vi "ReadTimeZoneCodes.vi"() -> (0 "x+y":dbl[](array[numeric])=[0.0, 1.0, 10.5, 9.5, -5.0, 10.5, 8.75, 3.0, -3.0, 11.0, 10.0, 11.0, 4.5, -8.0, -9.0, 6.0, -3.0, 5.0, -4.0, 4.0, 12.0, 12.0, 5.0, -3.0, 3.0, -4.0, -4.0, 9.0, 8.0, 0.0, -1.0, 5.0, 4.0, -12.0, 2.0, 8.0, -4.0, -2.0, -3.0, 6.0, 11.0, 1.0, 6.0, 3.0, 8.0, 2.0, 6.5, -5.0, -4.0, 2.0, 1.0, 13.75, 12.75, 9.0, 8.0, 8.0, 10.0, -4.0, -5.0, -10.0, -3.0, -3.0, -5.0, -6.0, 8.0, -5.0, -6.0, -1.0, 7.0, 10.0, 4.0, 7.0, 10.0, 5.0, -5.0, -5.0, 3.0, -5.0, -4.0, 3.0, 2.0, 0.0, -1.0, -5.0, -5.0, 6.0, 3.0, 13.0, 12.0, -3.0, -4.0, -2.0, 7.0, -6.0, -9.0, 4.0, -3.0, 12.0, 0.0, 4.0, -2.0, -4.0, 8.0, -9.0, -10.0, 8.0, 8.0, 7.0, 7.0, 9.0, 7.0, 3.0, 6.0, 4.5, 9.0, 8.0, 3.5, 5.5, 1.0, 2.0, 9.0, 10.0, 6.0, 11.0, 8.0, 7.0, 9.0, 4.0, 11.0, 11.0, 10.5, 14.0, 12.0, 12.0, 10.0, -8.5, 5.0, -6.0, 12.0, 6.5, 4.0, 3.0, -7.0, -7.0, 4.0, 5.0, 8.0, -1.0, 11.0, -1.5, 11.0, 7.0, 6.0, 5.75, 12.0, -2.5, -11.0, 13.0, 12.0, -2.0, 7.0, 6.0, 5.0, -3.0, -7.0, -5.0, 12.0, 12.0, 10.0, 13.0, 8.0, 5.0, -2.0, -3.0, 11.0, -8.0, -8.0, -8.0, 9.0, -3.0, -4.0, 8.5, 8.5, -4.0, 6.0, -5.0, 4.0, -3.0, -6.0, 10.0, 4.0, 2.0, 11.0, 4.0, 8.0, 11.0, -3.0, -11.0, 3.0, -7.0, -10.0, 5.0, 5.0, 13.0, 9.0, 5.0, 13.0, 12.0, -8.0, 9.0, 8.0, 8.0, 8.0, 0.0, -2.0, -3.0, 5.0, -9.0, -3.5, 11.0, 10.0, 6.0, 11.0, -10.0, 12.0, -3.0, 2.0, 1.0, 1.0, 0.0, 12.0, -2.0, -3.0, 7.0, 9.0, 8.0, 13.0, 1.0, 0.0, -11.0, -12.0, 10.0, 9.0, 10.0, 6.0, 5.0, 0.0], 1 "Abbreviation":string[](array[string])=["Abbreviation", "A", "ACDT", "ACST", "ACT", "ACT", "ACWST", "ADT", "ADT", "AEDT", "AEST", "AET", "AFT", "AKDT", "AKST", "ALMT", "AMST", "AMST", "AMT", "AMT", "ANAST", "ANAT", "AQTT", "ART", "AST", "AST", "AT", "AWDT", "AWST", "AZOST", "AZOT", "AZST", "AZT", "AoE", "B", "BNT", "BOT", "BRST", "BRT", "BST", "BST", "BST", "BTT", "C", "CAST", "CAT", "CCT", "CDT", "CDT", "CEST", "CET", "CHADT", "CHAST", "CHOST", "CHOST", "CHOT", "CHUT", "CIDST", "CIST", "CKT", "CLST", "CLT", "COT", "CST", "CST", "CST", "CT", "CVT", "CXT", "ChST", "D", "DAVT", "DDUT", "E", "EASST", "EAST", "EAT", "ECT", "EDT", "EEST", "EET", "EGST", "EGT", "EST", "ET", "F", "FET", "FJST", "FJT", "FKST", "FKT", "FNT", "G", "GALT", "GAMT", "GET", "GFT", "GILT", "GMT", "GST", "GST", "GYT", "H", "HADT", "HAST", "HKT", "HOVST", "HOVST", "HOVT", "I", "ICT", "IDT", "IOT", "IRDT", "IRKST", "IRKT", "IRST", "IST", "IST", "IST", "JST", "K", "KGT", "KOST", "KRAST", "KRAT", "KST", "KUYT", "L", "LHDT", "LHST", "LINT", "M", "MAGST", "MAGT", "MART", "MAWT", "MDT", "MHT", "MMT", "MSD", "MSK", "MST", "MT", "MUT", "MVT", "MYT", "N", "NCT", "NDT", "NFT", "NOVST", "NOVT", "NPT", "NRT", "NST", "NUT", "NZDT", "NZST", "O", "OMSST", "OMST", "ORAT", "P", "PDT", "PET", "PETST", "PETT", "PGT", "PHOT", "PHT", "PKT", "PMDT", "PMST", "PONT", "PST", "PST", "PT", "PWT", "PYST", "PYT", "PYT", "PYT", "Q", "QYZT", "R", "RET", "ROTT", "S", "SAKT", "SAMT", "SAST", "SBT", "SCT", "SGT", "SRET", "SRT", "SST", "SYOT", "T", "TAHT", "TFT", "TJT", "TKT", "TLT", "TMT", "TOT", "TVT", "U", "ULAST", "ULAST", "ULAT", "ULAT", "UTC", "UYST", "UYT", "UZT", "V", "VET", "VLAST", "VLAT", "VOST", "VUT", "W", "WAKT", "WARST", "WAST", "WAT", "WEST", "WET", "WFT", "WGST", "WGT", "WIB", "WIT", "WITA", "WST", "WST", "WT", "X", "Y", "YAKST", "YAKT", "YAPT", "YEKST", "YEKT", "Z"])   [LabVIEW 2015]
doc: "In order to Read and Write to any of the numerous pre-configured LabJack T7 Registers, the expected data type needs to be identified. This VI parses the T7 MODBUS Map (.json file), and searches the array to identify the Data Type expected for a desired Register. It also returns the Register Name. Like Registers are grouped in the Map list (e.g. AIN#(0:254)), so if a Selected Register is not exactly matched, a nearest neighbor is sought toward -Inf, and the values of the Nearest Likely Register are returned."
uses:
  <vilib>/regexp/Match Regular Expression.xnode
panel:
  out "UTC Offset.m":string[](array[string])=["", "00", "30", "30", "00", "30 / +9", "45", "00", "00", "00", "00", "00 / +10", "30", "00", "00", "00", "00", "00", "00", "00", "00", "00", "00", "00", "00", "00", "00 / -3", "00", "00", "00", "00", "00", "00", "00", "00", "00", "00", "00", "00", "00", "00", "00", "00", "00", "00", "00", "30", "00", "00", "00", "00", "45", "45", "00", "00 / +9", "00", "00", "00", "00", "00", "00", "00", "00", "00", "00", "00", "00 / -5", "00", "00", "00", "00", "00", "00", "00", "00", "00", "00", "00", "00", "00", "00", "00", "00", "00", "00 / -4", "00", "00", "00", "00", "00", "00", "00", "00", "00", "00", "00", "00", "00", "00", "00", "00", "00", "00", "00", "00", "00", "00", "00 / +8", "00", "00", "00", "00", "00", "30", "00", "00", "30", "30", "00", "00", "00", "00", "00", "00", "00", "00", "00", "00", "00", "00", "30", "00", "00", "00", "00", "30", "00", "00", "00", "30", "00", "00", "00", "00 / -6", "00", "00", "00", "00", "00", "30", "00", "00", "00", "45", "00", "30", "00", "00", "00", "00", "00", "00", "00", "00", "00", "00", "00", "00", "00", "00", "00", "00", "00", "00", "00", "00", "00", "00 / -7", "00", "00", "00", "30", "30", "00", "00", "00", "00", "00", "00", "00", "00", "00", "00", "00", "00", "00", "00", "00", "00", "00", "00", "00", "00", "00", "00", "00", "00", "00", "00", "00", "00 / +9", "00", "00 / +9", "", "00", "00", "00", "00", "30", "00", "00", "00", "00", "00", "00", "00", "00", "00", "00", "00", "00", "00", "00", "00", "00", "00", "00", "00", "00", "00", "00", "00", "00", "00", "00", "00", "00"]
  out "text":string="Abbreviation\tTime Zone Name\tLocation\tOffset ( x)\nA\tAlpha Time Zone\tMilitary\t1:00\nACDT\tAustralian Central Daylight Time  CDT – Central Daylight Time CDST – Central Daylight Savings Time\tAustralia\t10:30\nACST\tAustralian Central Standard Time  CST – Central Standard Time\tAustralia\t9:30\nACT\tAcre Time\tSouth America\t-5:00:00\nACT\tAustralian Central Time\tAustralia\t10:30 / +9:30\nACWST\tAustralian Central Western Standard Time\tAustralia\t8:45\nADT\tArabia Daylight Time  AST – Arabia Summer Time\tAsia\t3:00\nADT\tAtlantic Daylight Time  ADST – Atlantic Daylight Saving Time AST – Atlantic Summer Time  HAA – Heure Avancée de l'Atlantique (French)\tNorth America Atlantic\t-3:00:00\nAEDT\tAustralian Eastern Daylight Time  EDT – Eastern Daylight Time EDST – Eastern Daylight Saving Time\tAustralia Pacific\t11:00\nAEST\tAustralian Eastern Standard Time  EST – Eastern Standard Time AET – Australian Eastern Time\tAustralia\t10:00\nAET\tAustralian Eastern Time\tAustralia Pacific\t11:00 / +10:00\nAFT\tAfghanistan Time\tAsia\t4:30\nAKDT\tAlaska Daylight Time  ADST – Alaska Daylight Saving Time\tNorth America\t-8:00:00\nAKST\tAlaska Standard Time  AT – Alaska Time\tNorth America\t-9:00:00\nALMT\tAlma-Ata Time\tAsia\t6:00\nAMST\tAmazon Summer Time\tSouth America\t-3:00:00\nAMST\tArmenia Summer Time  AMDT – Armenia Daylight Time\tAsia\t5:00\nAMT\tAmazon Time\tSouth America\t-4:00:00\nAMT\tArmenia Time\tAsia\t4:00\nANAST\tAnadyr Summer Time\tAsia\t12:00\nANAT\tAnadyr Time\tAsia\t12:00\nAQTT\tAqtobe Time\tAsia\t5:00\nART\tArgentina Time\tAntarctica South America\t-3:00:00\nAST\tArabia Standard Time  AST – Arabic Standard Time AST – Al Manamah Standard Time\tAsia\t3:00\nAST\tAtlantic Standard Time  AT – Atlantic Time  AST – Tiempo Estándar del Atlántico (Spanish) HNA – Heure Normale de l'Atlantique (French)\tNorth America Atlantic Caribbean\t-4:00:00\nAT\tAtlantic Time\tNorth America Atlantic Caribbean\t-4:00 / -3:00\nAWDT\tAustralian Western Daylight Time  WDT – Western Daylight Time WST – Western Summer Time\tAustralia\t9:00\nAWST\tAustralian Western Standard Time  WST – Western Standard Time WAT – Western Australia Time\tAustralia\t8:00\nAZOST\tAzores Summer Time  AZODT – Azores Daylight Time\tAtlantic\t0:00\nAZOT\tAzores Time  AZOST – Azores Standard Time\tAtlantic\t-1:00:00\nAZST\tAzerbaijan Summer Time\tAsia\t5:00\nAZT\tAzerbaijan Time\tAsia\t4:00\nAoE\tAnywhere on Earth\tPacific\t-12:00:00\nB\tBravo Time Zone\tMilitary\t2:00\nBNT\tBrunei Darussalam Time  BDT – Brunei Time\tAsia\t8:00\nBOT\tBolivia Time\tSouth America\t-4:00:00\nBRST\tBrasília Summer Time  BST – Brazil Summer Time BST – Brazilian Summer Time\tSouth America\t-2:00:00\nBRT\tBrasília Time  BT – Brazil Time BT – Brazilian Time\tSouth America\t-3:00:00\nBST\tBangladesh Standard Time\tAsia\t6:00\nBST\tBougainville Standard Time\tPacific\t11:00\nBST\tBritish Summer Time  BDT – British Daylight Time BDST – British Daylight Saving Time\tEurope\t1:00\nBTT\tBhutan Time\tAsia\t6:00\nC\tCharlie Time Zone\tMilitary\t3:00\nCAST\tCasey Time\tAntarctica\t8:00\nCAT\tCentral Africa Time\tAfrica\t2:00\nCCT\tCocos Islands Time\tIndian Ocean\t6:30\nCDT\tCentral Daylight Time  CDST – Central Daylight Saving Time NACDT – North American Central Daylight Time  HAC – Heure Avancée du Centre (French)\tNorth America\t-5:00:00\nCDT\tCuba Daylight Time\tCaribbean\t-4:00:00\nCEST\tCentral European Summer Time  CEDT – Central European Daylight Time ECST – European Central Summer Time  MESZ – Mitteleuropäische Sommerzeit (German)\tEurope Antarctica\t2:00\nCET\tCentral European Time  ECT – European Central Time CET – Central Europe Time  MEZ – Mitteleuropäische Zeit (German)\tEurope Africa Antarctica\t1:00\nCHADT\tChatham Island Daylight Time  CDT – Chatham Daylight Time\tPacific\t13:45\nCHAST\tChatham Island Standard Time\tPacific\t12:45\nCHOST\tChoibalsan Summer Time  CHODT – Choibalsan Daylight Time CHODST – Choibalsan Daylight Saving Time\tAsia\t9:00\nCHOST\tChoibalsan Summer Time\tAsia\t8:00 / +9:00\nCHOT\tChoibalsan Time\tAsia\t8:00\nCHUT\tChuuk Time\tPacific\t10:00\nCIDST\tCayman Islands Daylight Saving Time\tCaribbean\t-4:00:00\nCIST\tCayman Islands Standard Time  CIT – Cayman Islands Time\tCaribbean\t-5:00:00\nCKT\tCook Island Time\tPacific\t-10:00:00\nCLST\tChile Summer Time  CLDT – Chile Daylight Time\tSouth America Antarctica\t-3:00:00\nCLT\tChile Standard Time  CT – Chile Time CLST – Chile Standard Time\tSouth America Antarctica\t-3:00:00\nCOT\tColombia Time\tSouth America\t-5:00:00\nCST\tCentral Standard Time  CT – Central Time NACST – North American Central Standard Time  CST – Tiempo Central Estándar (Spanish) HNC – Heure Normale du Centre (French)\tNorth America Central America\t-6:00:00\nCST\tChina Standard Time\tAsia\t8:00\nCST\tCuba Standard Time\tCaribbean\t-5:00:00\nCT\tCentral Time\tNorth America Central America\t-6:00 / -5:00\nCVT\tCape Verde Time\tAfrica\t-1:00:00\nCXT\tChristmas Island Time\tAustralia\t7:00\nChST\tChamorro Standard Time  GST – Guam Standard Time\tPacific\t10:00\nD\tDelta Time Zone\tMilitary\t4:00\nDAVT\tDavis Time\tAntarctica\t7:00\nDDUT\tDumont-d'Urville Time\tAntarctica\t10:00\nE\tEcho Time Zone\tMilitary\t5:00\nEASST\tEaster Island Summer Time  EADT – Easter Island Daylight Time\tPacific\t-5:00:00\nEAST\tEaster Island Standard Time\tPacific\t-5:00:00\nEAT\tEastern Africa Time  EAT – East Africa Time\tAfrica Indian Ocean\t3:00\nECT\tEcuador Time\tSouth America\t-5:00:00\nEDT\tEastern Daylight Time  EDST – Eastern Daylight Savings Time NAEDT – North American Eastern Daylight Time  HAE – Heure Avancée de l'Est (French) EDT – Tiempo de verano del Este (Spanish)\tNorth America Caribbean\t-4:00:00\nEEST\tEastern European Summer Time  EEDT – Eastern European Daylight Time  OESZ – Osteuropäische Sommerzeit (German)\tEurope Asia\t3:00\nEET\tEastern European Time  OEZ – Osteuropäische Zeit (German)\tEurope Asia Africa\t2:00\nEGST\tEastern Greenland Summer Time  EGST – East Greenland Summer Time\tNorth America\t0:00\nEGT\tEast Greenland Time  EGT – Eastern Greenland Time\tNorth America\t-1:00:00\nEST\tEastern Standard Time  ET – Eastern Time  NAEST – North American Eastern Standard Time  ET – Tiempo del Este (Spanish) HNE – Heure Normale de l'Est (French)\tNorth America Caribbean Central America\t-5:00:00\nET\tEastern Time\tNorth America Caribbean Central America\t-5:00 / -4:00\nF\tFoxtrot Time Zone\tMilitary\t6:00\nFET\tFurther-Eastern European Time\tEurope\t3:00\nFJST\tFiji Summer Time  FJDT – Fiji Daylight Time\tPacific\t13:00\nFJT\tFiji Time\tPacific\t12:00\nFKST\tFalkland Islands Summer Time  FKDT – Falkland Island Daylight Time\tSouth America\t-3:00:00\nFKT\tFalkland Island Time  FKST – Falkland Island Standard Time\tSouth America\t-4:00:00\nFNT\tFernando de Noronha Time\tSouth America\t-2:00:00\nG\tGolf Time Zone\tMilitary\t7:00\nGALT\tGalapagos Time\tPacific\t-6:00:00\nGAMT\tGambier Time  GAMT – Gambier Islands Time\tPacific\t-9:00:00\nGET\tGeorgia Standard Time\tAsia\t4:00\nGFT\tFrench Guiana Time\tSouth America\t-3:00:00\nGILT\tGilbert Island Time\tPacific\t12:00\nGMT\tGreenwich Mean Time  \"– Coordinated Universal Time GT – Greenwich Time\tEurope Africa North America Antarctica\t0:00\nGST\tGulf Standard Time\tAsia\t4:00\nGST\tSouth Georgia Time\tSouth America\t-2:00:00\nGYT\tGuyana Time\tSouth America\t-4:00:00\nH\tHotel Time Zone\tMilitary\t8:00\nHADT\tHawaii-Aleutian Daylight Time  HDT – Hawaii Daylight Time\tNorth America\t-9:00:00\nHAST\tHawaii-Aleutian Standard Time  HST – Hawaii Standard Time\tNorth America Pacific\t-10:00:00\nHKT\tHong Kong Time\tAsia\t8:00\nHOVST\tHovd Summer Time  HOVDT – Hovd Daylight Time HOVDST – Hovd Daylight Saving Time\tAsia\t8:00\nHOVST\tHovd Summer Time\tAsia\t7:00 / +8:00\nHOVT\tHovd Time\tAsia\t7:00\nI\tIndia Time Zone\tMilitary\t9:00\nICT\tIndochina Time\tAsia\t7:00\nIDT\tIsrael Daylight Time\tAsia\t3:00\nIOT\tIndian Chagos Time\tIndian Ocean\t6:00\nIRDT\tIran Daylight Time  IRST – Iran Summer Time IDT – Iran Daylight Time\tAsia\t4:30\nIRKST\tIrkutsk Summer Time\tAsia\t9:00\nIRKT\tIrkutsk Time\tAsia\t8:00\nIRST\tIran Standard Time  IT – Iran Time\tAsia\t3:30\nIST\tIndia Standard Time  IT – India Time IST – Indian Standard Time\tAsia\t5:30\nIST\tIrish Standard Time  IST – Irish Summer Time\tEurope\t1:00\nIST\tIsrael Standard Time\tAsia\t2:00\nJST\tJapan Standard Time\tAsia\t9:00\nK\tKilo Time Zone\tMilitary\t10:00\nKGT\tKyrgyzstan Time\tAsia\t6:00\nKOST\tKosrae Time\tPacific\t11:00\nKRAST\tKrasnoyarsk Summer Time\tAsia\t8:00\nKRAT\tKrasnoyarsk Time\tAsia\t7:00\nKST\tKorea Standard Time  KST – Korean Standard Time KT – Korea Time\tAsia\t9:00\nKUYT\tKuybyshev Time  SAMST – Samara Summer Time\tEurope\t4:00\nL\tLima Time Zone\tMilitary\t11:00\nLHDT\tLord Howe Daylight Time\tAustralia\t11:00\nLHST\tLord Howe Standard Time\tAustralia\t10:30\nLINT\tLine Islands Time\tPacific\t14:00\nM\tMike Time Zone\tMilitary\t12:00\nMAGST\tMagadan Summer Time  MAGST – Magadan Island Summer Time\tAsia\t12:00\nMAGT\tMagadan Time  MAGT – Magadan Island Time\tAsia\t10:00\nMART\tMarquesas Time\tPacific\t-9:30:00\nMAWT\tMawson Time\tAntarctica\t5:00\nMDT\tMountain Daylight Time  MDST – Mountain Daylight Saving Time NAMDT – North American Mountain Daylight Time  HAR – Heure Avancée des Rocheuses (French)\tNorth America\t-6:00:00\nMHT\tMarshall Islands Time\tPacific\t12:00\nMMT\tMyanmar Time\tAsia\t6:30\nMSD\tMoscow Daylight Time  Moscow Summer Time\tEurope\t4:00\nMSK\tMoscow Standard Time  MCK – Moscow Time\tEurope Asia\t3:00\nMST\tMountain Standard Time  MT – Mountain Time NAMST – North American Mountain Standard Time  HNR – Heure Normale des Rocheuses (French)\tNorth America\t-7:00:00\nMT\tMountain Time\tNorth America\t-7:00 / -6:00\nMUT\tMauritius Time\tAfrica\t4:00\nMVT\tMaldives Time\tAsia\t5:00\nMYT\tMalaysia Time  MST – Malaysian Standard Time\tAsia\t8:00\nN\tNovember Time Zone\tMilitary\t-1:00:00\nNCT\tNew Caledonia Time\tPacific\t11:00\nNDT\tNewfoundland Daylight Time  HAT – Heure Avancée de Terre-Neuve (French)\tNorth America\t-2:30:00\nNFT\tNorfolk Time  NFT – Norfolk Island Time\tAustralia\t11:00\nNOVST\tNovosibirsk Summer Time  OMSST – Omsk Summer Time\tAsia\t7:00\nNOVT\tNovosibirsk Time  OMST – Omsk Standard Time\tAsia\t6:00\nNPT\tNepal Time\tAsia\t5:45\nNRT\tNauru Time\tPacific\t12:00\nNST\tNewfoundland Standard Time  HNT – Heure Normale de Terre-Neuve (French)\tNorth America\t-3:30:00\nNUT\tNiue Time\tPacific\t-11:00:00\nNZDT\tNew Zealand Daylight Time\tPacific Antarctica\t13:00\nNZST\tNew Zealand Standard Time\tPacific Antarctica\t12:00\nO\tOscar Time Zone\tMilitary\t-2:00:00\nOMSST\tOmsk Summer Time  NOVST – Novosibirsk Summer Time\tAsia\t7:00\nOMST\tOmsk Standard Time  OMST – Omsk Time NOVT – Novosibirsk Time\tAsia\t6:00\nORAT\tOral Time\tAsia\t5:00\nP\tPapa Time Zone\tMilitary\t-3:00:00\nPDT\tPacific Daylight Time  PDST – Pacific Daylight Saving Time NAPDT – North American Pacific Daylight Time  HAP – Heure Avancée du Pacifique (French)\tNorth America\t-7:00:00\nPET\tPeru Time\tSouth America\t-5:00:00\nPETST\tKamchatka Summer Time\tAsia\t12:00\nPETT\tKamchatka Time  PETT – Petropavlovsk-Kamchatski Time\tAsia\t12:00\nPGT\tPapua New Guinea Time\tPacific\t10:00\nPHOT\tPhoenix Island Time\tPacific\t13:00\nPHT\tPhilippine Time  PST – Philippine Standard Time\tAsia\t8:00\nPKT\tPakistan Standard Time  PKT – Pakistan Time\tAsia\t5:00\nPMDT\tPierre & Miquelon Daylight Time\tNorth America\t-2:00:00\nPMST\tPierre & Miquelon Standard Time\tNorth America\t-3:00:00\nPONT\tPohnpei Standard Time\tPacific\t11:00\nPST\tPacific Standard Time  PT – Pacific Time NAPST – North American Pacific Standard Time  PT – Tiempo del Pacífico (Spanish) HNP – Heure Normale du Pacifique (French)\tNorth America\t-8:00:00\nPST\tPitcairn Standard Time\tPacific\t-8:00:00\nPT\tPacific Time\tNorth America\t-8:00 / -7:00\nPWT\tPalau Time\tPacific\t9:00\nPYST\tParaguay Summer Time\tSouth America\t-3:00:00\nPYT\tParaguay Time\tSouth America\t-4:00:00\nPYT\tPyongyang Time  PYST – Pyongyang Standard Time\tAsia\t8:30\nPYT\tPyongyang Time\tAsia\t8:30\nQ\tQuebec Time Zone\tMilitary\t-4:00:00\nQYZT\tQyzylorda Time\tAsia\t6:00\nR\tRomeo Time Zone\tMilitary\t-5:00:00\nRET\tReunion Time\tAfrica\t4:00\nROTT\tRothera Time\tAntarctica\t-3:00:00\nS\tSierra Time Zone\tMilitary\t-6:00:00\nSAKT\tSakhalin Time\tAsia\t10:00\nSAMT\tSamara Time  SAMT – Samara Standard Time\tEurope\t4:00\nSAST\tSouth Africa Standard Time  SAST – South African Standard Time\tAfrica\t2:00\nSBT\tSolomon Islands Time  SBT – Solomon Island Time\tPacific\t11:00\nSCT\tSeychelles Time\tAfrica\t4:00\nSGT\tSingapore Time  SST – Singapore Standard Time\tAsia\t8:00\nSRET\tSrednekolymsk Time\tAsia\t11:00\nSRT\tSuriname Time\tSouth America\t-3:00:00\nSST\tSamoa Standard Time\tPacific\t-11:00:00\nSYOT\tSyowa Time\tAntarctica\t3:00\nT\tTango Time Zone\tMilitary\t-7:00:00\nTAHT\tTahiti Time\tPacific\t-10:00:00\nTFT\tFrench Southern and Antarctic Time  KIT – Kerguelen (Islands) Time\tIndian Ocean\t5:00\nTJT\tTajikistan Time\tAsia\t5:00\nTKT\tTokelau Time\tPacific\t13:00\nTLT\tEast Timor Time\tAsia\t9:00\nTMT\tTurkmenistan Time\tAsia\t5:00\nTOT\tTonga Time\tPacific\t13:00\nTVT\tTuvalu Time\tPacific\t12:00\nU\tUniform Time Zone\tMilitary\t-8:00:00\nULAST\tUlaanbaatar Summer Time  ULAST – Ulan Bator Summer Time\tAsia\t9:00\nULAST\tUlaanbaatar Summer Time\tAsia\t8:00 / +9:00\nULAT\tUlaanbaatar Time  ULAT – Ulan Bator Time\tAsia\t8:00\nULAT\tUlaanbaatar Time\tAsia\t8:00 / +9:00\nUTC\tCoordinated Universal Time\tWorldwide\tUTC\nUYST\tUruguay Summer Time\tSouth America\t-2:00:00\nUYT\tUruguay Time\tSouth America\t-3:00:00\nUZT\tUzbekistan Time\tAsia\t5:00\nV\tVictor Time Zone\tMilitary\t-9:00:00\nVET\tVenezuelan Standard Time  HLV – Hora Legal de Venezuela (Spanish)\tSouth America\t-4:30:00\nVLAST\tVladivostok Summer Time\tAsia\t11:00\nVLAT\tVladivostok Time\tAsia\t10:00\nVOST\tVostok Time\tAntarctica\t6:00\nVUT\tVanuatu Time  EFATE – Efate Time\tPacific\t11:00\nW\tWhiskey Time Zone\tMilitary\t-10:00:00\nWAKT\tWake Time\tPacific\t12:00\nWARST\tWestern Argentine Summer Time\tSouth America\t-3:00:00\nWAST\tWest Africa Summer Time\tAfrica\t2:00\nWAT\tWest Africa Time\tAfrica\t1:00\nWEST\tWestern European Summer Time  WEDT – Western European Daylight Time  WESZ – Westeuropäische Sommerzeit (German)\tEurope Africa\t1:00\nWET\tWestern European Time  GMT – Greenwich Mean Time  WEZ – Westeuropäische Zeit (German)\tEurope Africa\t0:00\nWFT\tWallis and Futuna Time\tPacific\t12:00\nWGST\tWestern Greenland Summer Time  WGST – West Greenland Summer Time\tNorth America\t-2:00:00\nWGT\tWest Greenland Time  WGT – Western Greenland Time\tNorth America\t-3:00:00\nWIB\tWestern Indonesian Time  WIB – Waktu Indonesia Barat\tAsia\t7:00\nWIT\tEastern Indonesian Time  WIT – Waktu Indonesia Timur\tAsia\t9:00\nWITA\tCentral Indonesian Time  WITA – Waktu Indonesia Tengah\tAsia\t8:00\nWST\tWest Samoa Time  ST – Samoa Time\tPacific\t13:00\nWST\tWestern Sahara Summer Time\tAfrica\t1:00\nWT\tWestern Sahara Standard Time  WT – Western Sahara Time\tAfrica\t0:00\nX\tX-ray Time Zone\tMilitary\t-11:00:00\nY\tYankee Time Zone\tMilitary\t-12:00:00\nYAKST\tYakutsk Summer Time\tAsia\t10:00\nYAKT\tYakutsk Time\tAsia\t9:00\nYAPT\tYap Time\tPacific\t10:00\nYEKST\tYekaterinburg Summer Time\tAsia\t6:00\nYEKT\tYekaterinburg Time\tAsia\t5:00\nZ\tZulu Time Zone\tMilitary\t0:00"
  out "Location":string[](array[string])=["Location", "Military", "Australia", "Australia", "South America", "Australia", "Australia", "Asia", "North America Atlantic", "Australia Pacific", "Australia", "Australia Pacific", "Asia", "North America", "North America", "Asia", "South America", "Asia", "South America", "Asia", "Asia", "Asia", "Asia", "Antarctica South America", "Asia", "North America Atlantic Caribbean", "North America Atlantic Caribbean", "Australia", "Australia", "Atlantic", "Atlantic", "Asia", "Asia", "Pacific", "Military", "Asia", "South America", "South America", "South America", "Asia", "Pacific", "Europe", "Asia", "Military", "Antarctica", "Africa", "Indian Ocean", "North America", "Caribbean", "Europe Antarctica", "Europe Africa Antarctica", "Pacific", "Pacific", "Asia", "Asia", "Asia", "Pacific", "Caribbean", "Caribbean", "Pacific", "South America Antarctica", "South America Antarctica", "South America", "North America Central America", "Asia", "Caribbean", "North America Central America", "Africa", "Australia", "Pacific", "Military", "Antarctica", "Antarctica", "Military", "Pacific", "Pacific", "Africa Indian Ocean", "South America", "North America Caribbean", "Europe Asia", "Europe Asia Africa", "North America", "North America", "North America Caribbean Central America", "North America Caribbean Central America", "Military", "Europe", "Pacific", "Pacific", "South America", "South America", "South America", "Military", "Pacific", "Pacific", "Asia", "South America", "Pacific", "Europe Africa North America Antarctica", "Asia", "South America", "South America", "Military", "North America", "North America Pacific", "Asia", "Asia", "Asia", "Asia", "Military", "Asia", "Asia", "Indian Ocean", "Asia", "Asia", "Asia", "Asia", "Asia", "Europe", "Asia", "Asia", "Military", "Asia", "Pacific", "Asia", "Asia", "Asia", "Europe", "Military", "Australia", "Australia", "Pacific", "Military", "Asia", "Asia", "Pacific", "Antarctica", "North America", "Pacific", "Asia", "Europe", "Europe Asia", "North America", "North America", "Africa", "Asia", "Asia", "Military", "Pacific", "North America", "Australia", "Asia", "Asia", "Asia", "Pacific", "North America", "Pacific", "Pacific Antarctica", "Pacific Antarctica", "Military", "Asia", "Asia", "Asia", "Military", "North America", "South America", "Asia", "Asia", "Pacific", "Pacific", "Asia", "Asia", "North America", "North America", "Pacific", "North America", "Pacific", "North America", "Pacific", "South America", "South America", "Asia", "Asia", "Military", "Asia", "Military", "Africa", "Antarctica", "Military", "Asia", "Europe", "Africa", "Pacific", "Africa", "Asia", "Asia", "South America", "Pacific", "Antarctica", "Military", "Pacific", "Indian Ocean", "Asia", "Pacific", "Asia", "Asia", "Pacific", "Pacific", "Military", "Asia", "Asia", "Asia", "Asia", "Worldwide", "South America", "South America", "Asia", "Military", "South America", "Asia", "Asia", "Antarctica", "Pacific", "Military", "Pacific", "South America", "Africa", "Africa", "Europe Africa", "Europe Africa", "Pacific", "North America", "North America", "Asia", "Asia", "Asia", "Pacific", "Africa", "Africa", "Military", "Military", "Asia", "Asia", "Pacific", "Asia", "Asia", "Military"]
  out "UTC Offset.h":string[](array[string])=["Offset ( x)", "1", "10", "9", "-5", "10", "8", "3", "-3", "11", "10", "11", "4", "-8", "-9", "6", "-3", "5", "-4", "4", "12", "12", "5", "-3", "3", "-4", "-4", "9", "8", "0", "-1", "5", "4", "-12", "2", "8", "-4", "-2", "-3", "6", "11", "1", "6", "3", "8", "2", "6", "-5", "-4", "2", "1", "13", "12", "9", "8", "8", "10", "-4", "-5", "-10", "-3", "-3", "-5", "-6", "8", "-5", "-6", "-1", "7", "10", "4", "7", "10", "5", "-5", "-5", "3", "-5", "-4", "3", "2", "0", "-1", "-5", "-5", "6", "3", "13", "12", "-3", "-4", "-2", "7", "-6", "-9", "4", "-3", "12", "0", "4", "-2", "-4", "8", "-9", "-10", "8", "8", "7", "7", "9", "7", "3", "6", "4", "9", "8", "3", "5", "1", "2", "9", "10", "6", "11", "8", "7", "9", "4", "11", "11", "10", "14", "12", "12", "10", "-9", "5", "-6", "12", "6", "4", "3", "-7", "-7", "4", "5", "8", "-1", "11", "-2", "11", "7", "6", "5", "12", "-3", "-11", "13", "12", "-2", "7", "6", "5", "-3", "-7", "-5", "12", "12", "10", "13", "8", "5", "-2", "-3", "11", "-8", "-8", "-8", "9", "-3", "-4", "8", "8", "-4", "6", "-5", "4", "-3", "-6", "10", "4", "2", "11", "4", "8", "11", "-3", "-11", "3", "-7", "-10", "5", "5", "13", "9", "5", "13", "12", "-8", "9", "8", "8", "8", "UTC", "-2", "-3", "5", "-9", "-4", "11", "10", "6", "11", "-10", "12", "-3", "2", "1", "1", "0", "12", "-2", "-3", "7", "9", "8", "13", "1", "0", "-11", "-12", "10", "9", "10", "6", "5", "0"]
  out "Time Zone Name":string[](array[string])=["Time Zone Name", "Alpha Time Zone", "Australian Central Daylight Time  CDT – Central Daylight Time CDST – Central Daylight Savings Time", "Australian Central Standard Time  CST – Central Standard Time", "Acre Time", "Australian Central Time", "Australian Central Western Standard Time", "Arabia Daylight Time  AST – Arabia Summer Time", "Atlantic Daylight Time  ADST – Atlantic Daylight Saving Time AST – Atlantic Summer Time  HAA – Heure Avancée de l'Atlantique (French)", "Australian Eastern Daylight Time  EDT – Eastern Daylight Time EDST – Eastern Daylight Saving Time", "Australian Eastern Standard Time  EST – Eastern Standard Time AET – Australian Eastern Time", "Australian Eastern Time", "Afghanistan Time", "Alaska Daylight Time  ADST – Alaska Daylight Saving Time", "Alaska Standard Time  AT – Alaska Time", "Alma-Ata Time", "Amazon Summer Time", "Armenia Summer Time  AMDT – Armenia Daylight Time", "Amazon Time", "Armenia Time", "Anadyr Summer Time", "Anadyr Time", "Aqtobe Time", "Argentina Time", "Arabia Standard Time  AST – Arabic Standard Time AST – Al Manamah Standard Time", "Atlantic Standard Time  AT – Atlantic Time  AST – Tiempo Estándar del Atlántico (Spanish) HNA – Heure Normale de l'Atlantique (French)", "Atlantic Time", "Australian Western Daylight Time  WDT – Western Daylight Time WST – Western Summer Time", "Australian Western Standard Time  WST – Western Standard Time WAT – Western Australia Time", "Azores Summer Time  AZODT – Azores Daylight Time", "Azores Time  AZOST – Azores Standard Time", "Azerbaijan Summer Time", "Azerbaijan Time", "Anywhere on Earth", "Bravo Time Zone", "Brunei Darussalam Time  BDT – Brunei Time", "Bolivia Time", "Brasília Summer Time  BST – Brazil Summer Time BST – Brazilian Summer Time", "Brasília Time  BT – Brazil Time BT – Brazilian Time", "Bangladesh Standard Time", "Bougainville Standard Time", "British Summer Time  BDT – British Daylight Time BDST – British Daylight Saving Time", "Bhutan Time", "Charlie Time Zone", "Casey Time", "Central Africa Time", "Cocos Islands Time", "Central Daylight Time  CDST – Central Daylight Saving Time NACDT – North American Central Daylight Time  HAC – Heure Avancée du Centre (French)", "Cuba Daylight Time", "Central European Summer Time  CEDT – Central European Daylight Time ECST – European Central Summer Time  MESZ – Mitteleuropäische Sommerzeit (German)", "Central European Time  ECT – European Central Time CET – Central Europe Time  MEZ – Mitteleuropäische Zeit (German)", "Chatham Island Daylight Time  CDT – Chatham Daylight Time", "Chatham Island Standard Time", "Choibalsan Summer Time  CHODT – Choibalsan Daylight Time CHODST – Choibalsan Daylight Saving Time", "Choibalsan Summer Time", "Choibalsan Time", "Chuuk Time", "Cayman Islands Daylight Saving Time", "Cayman Islands Standard Time  CIT – Cayman Islands Time", "Cook Island Time", "Chile Summer Time  CLDT – Chile Daylight Time", "Chile Standard Time  CT – Chile Time CLST – Chile Standard Time", "Colombia Time", "Central Standard Time  CT – Central Time NACST – North American Central Standard Time  CST – Tiempo Central Estándar (Spanish) HNC – Heure Normale du Centre (French)", "China Standard Time", "Cuba Standard Time", "Central Time", "Cape Verde Time", "Christmas Island Time", "Chamorro Standard Time  GST – Guam Standard Time", "Delta Time Zone", "Davis Time", "Dumont-d'Urville Time", "Echo Time Zone", "Easter Island Summer Time  EADT – Easter Island Daylight Time", "Easter Island Standard Time", "Eastern Africa Time  EAT – East Africa Time", "Ecuador Time", "Eastern Daylight Time  EDST – Eastern Daylight Savings Time NAEDT – North American Eastern Daylight Time  HAE – Heure Avancée de l'Est (French) EDT – Tiempo de verano del Este (Spanish)", "Eastern European Summer Time  EEDT – Eastern European Daylight Time  OESZ – Osteuropäische Sommerzeit (German)", "Eastern European Time  OEZ – Osteuropäische Zeit (German)", "Eastern Greenland Summer Time  EGST – East Greenland Summer Time", "East Greenland Time  EGT – Eastern Greenland Time", "Eastern Standard Time  ET – Eastern Time  NAEST – North American Eastern Standard Time  ET – Tiempo del Este (Spanish) HNE – Heure Normale de l'Est (French)", "Eastern Time", "Foxtrot Time Zone", "Further-Eastern European Time", "Fiji Summer Time  FJDT – Fiji Daylight Time", "Fiji Time", "Falkland Islands Summer Time  FKDT – Falkland Island Daylight Time", "Falkland Island Time  FKST – Falkland Island Standard Time", "Fernando de Noronha Time", "Golf Time Zone", "Galapagos Time", "Gambier Time  GAMT – Gambier Islands Time", "Georgia Standard Time", "French Guiana Time", "Gilbert Island Time", "Greenwich Mean Time  \"– Coordinated Universal Time GT – Greenwich Time", "Gulf Standard Time", "South Georgia Time", "Guyana Time", "Hotel Time Zone", "Hawaii-Aleutian Daylight Time  HDT – Hawaii Daylight Time", "Hawaii-Aleutian Standard Time  HST – Hawaii Standard Time", "Hong Kong Time", "Hovd Summer Time  HOVDT – Hovd Daylight Time HOVDST – Hovd Daylight Saving Time", "Hovd Summer Time", "Hovd Time", "India Time Zone", "Indochina Time", "Israel Daylight Time", "Indian Chagos Time", "Iran Daylight Time  IRST – Iran Summer Time IDT – Iran Daylight Time", "Irkutsk Summer Time", "Irkutsk Time", "Iran Standard Time  IT – Iran Time", "India Standard Time  IT – India Time IST – Indian Standard Time", "Irish Standard Time  IST – Irish Summer Time", "Israel Standard Time", "Japan Standard Time", "Kilo Time Zone", "Kyrgyzstan Time", "Kosrae Time", "Krasnoyarsk Summer Time", "Krasnoyarsk Time", "Korea Standard Time  KST – Korean Standard Time KT – Korea Time", "Kuybyshev Time  SAMST – Samara Summer Time", "Lima Time Zone", "Lord Howe Daylight Time", "Lord Howe Standard Time", "Line Islands Time", "Mike Time Zone", "Magadan Summer Time  MAGST – Magadan Island Summer Time", "Magadan Time  MAGT – Magadan Island Time", "Marquesas Time", "Mawson Time", "Mountain Daylight Time  MDST – Mountain Daylight Saving Time NAMDT – North American Mountain Daylight Time  HAR – Heure Avancée des Rocheuses (French)", "Marshall Islands Time", "Myanmar Time", "Moscow Daylight Time  Moscow Summer Time", "Moscow Standard Time  MCK – Moscow Time", "Mountain Standard Time  MT – Mountain Time NAMST – North American Mountain Standard Time  HNR – Heure Normale des Rocheuses (French)", "Mountain Time", "Mauritius Time", "Maldives Time", "Malaysia Time  MST – Malaysian Standard Time", "November Time Zone", "New Caledonia Time", "Newfoundland Daylight Time  HAT – Heure Avancée de Terre-Neuve (French)", "Norfolk Time  NFT – Norfolk Island Time", "Novosibirsk Summer Time  OMSST – Omsk Summer Time", "Novosibirsk Time  OMST – Omsk Standard Time", "Nepal Time", "Nauru Time", "Newfoundland Standard Time  HNT – Heure Normale de Terre-Neuve (French)", "Niue Time", "New Zealand Daylight Time", "New Zealand Standard Time", "Oscar Time Zone", "Omsk Summer Time  NOVST – Novosibirsk Summer Time", "Omsk Standard Time  OMST – Omsk Time NOVT – Novosibirsk Time", "Oral Time", "Papa Time Zone", "Pacific Daylight Time  PDST – Pacific Daylight Saving Time NAPDT – North American Pacific Daylight Time  HAP – Heure Avancée du Pacifique (French)", "Peru Time", "Kamchatka Summer Time", "Kamchatka Time  PETT – Petropavlovsk-Kamchatski Time", "Papua New Guinea Time", "Phoenix Island Time", "Philippine Time  PST – Philippine Standard Time", "Pakistan Standard Time  PKT – Pakistan Time", "Pierre & Miquelon Daylight Time", "Pierre & Miquelon Standard Time", "Pohnpei Standard Time", "Pacific Standard Time  PT – Pacific Time NAPST – North American Pacific Standard Time  PT – Tiempo del Pacífico (Spanish) HNP – Heure Normale du Pacifique (French)", "Pitcairn Standard Time", "Pacific Time", "Palau Time", "Paraguay Summer Time", "Paraguay Time", "Pyongyang Time  PYST – Pyongyang Standard Time", "Pyongyang Time", "Quebec Time Zone", "Qyzylorda Time", "Romeo Time Zone", "Reunion Time", "Rothera Time", "Sierra Time Zone", "Sakhalin Time", "Samara Time  SAMT – Samara Standard Time", "South Africa Standard Time  SAST – South African Standard Time", "Solomon Islands Time  SBT – Solomon Island Time", "Seychelles Time", "Singapore Time  SST – Singapore Standard Time", "Srednekolymsk Time", "Suriname Time", "Samoa Standard Time", "Syowa Time", "Tango Time Zone", "Tahiti Time", "French Southern and Antarctic Time  KIT – Kerguelen (Islands) Time", "Tajikistan Time", "Tokelau Time", "East Timor Time", "Turkmenistan Time", "Tonga Time", "Tuvalu Time", "Uniform Time Zone", "Ulaanbaatar Summer Time  ULAST – Ulan Bator Summer Time", "Ulaanbaatar Summer Time", "Ulaanbaatar Time  ULAT – Ulan Bator Time", "Ulaanbaatar Time", "Coordinated Universal Time", "Uruguay Summer Time", "Uruguay Time", "Uzbekistan Time", "Victor Time Zone", "Venezuelan Standard Time  HLV – Hora Legal de Venezuela (Spanish)", "Vladivostok Summer Time", "Vladivostok Time", "Vostok Time", "Vanuatu Time  EFATE – Efate Time", "Whiskey Time Zone", "Wake Time", "Western Argentine Summer Time", "West Africa Summer Time", "West Africa Time", "Western European Summer Time  WEDT – Western European Daylight Time  WESZ – Westeuropäische Sommerzeit (German)", "Western European Time  GMT – Greenwich Mean Time  WEZ – Westeuropäische Zeit (German)", "Wallis and Futuna Time", "Western Greenland Summer Time  WGST – West Greenland Summer Time", "West Greenland Time  WGT – Western Greenland Time", "Western Indonesian Time  WIB – Waktu Indonesia Barat", "Eastern Indonesian Time  WIT – Waktu Indonesia Timur", "Central Indonesian Time  WITA – Waktu Indonesia Tengah", "West Samoa Time  ST – Samoa Time", "Western Sahara Summer Time", "Western Sahara Standard Time  WT – Western Sahara Time", "X-ray Time Zone", "Yankee Time Zone", "Yakutsk Summer Time", "Yakutsk Time", "Yap Time", "Yekaterinburg Summer Time", "Yekaterinburg Time", "Zulu Time Zone"]
  in  "Time Zone Code Relative Path":path=path "Time Zone Codes.xls"
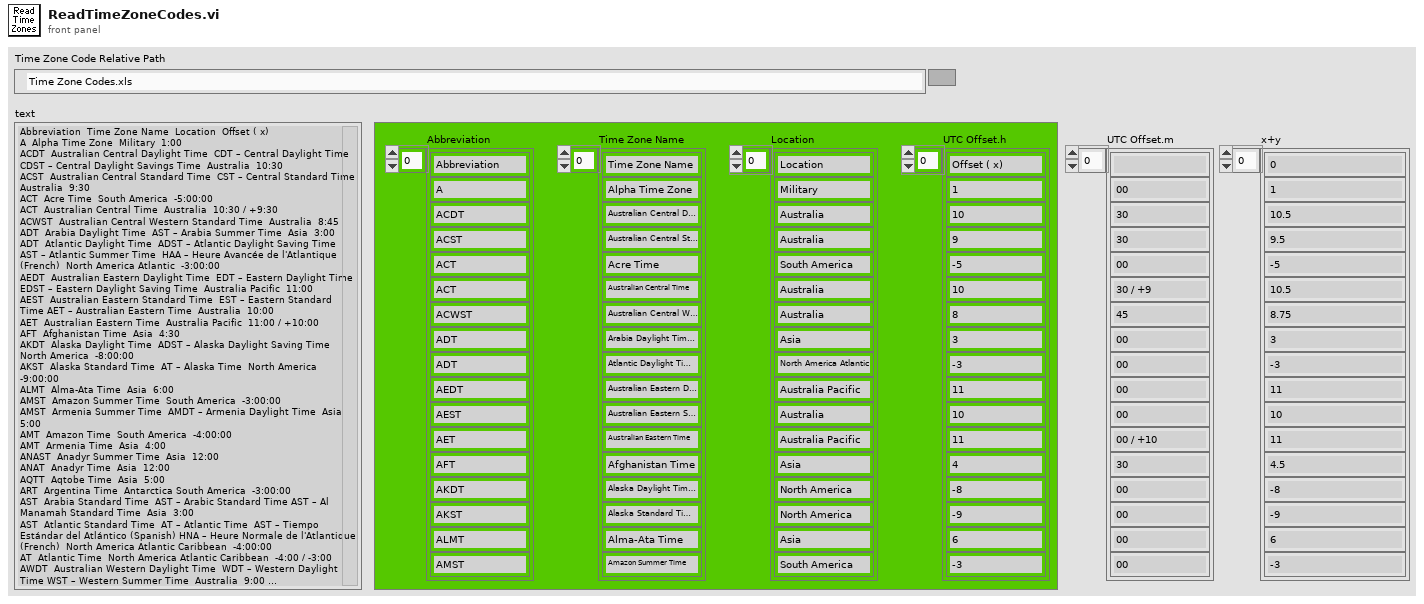
[diagram p1: front panel]
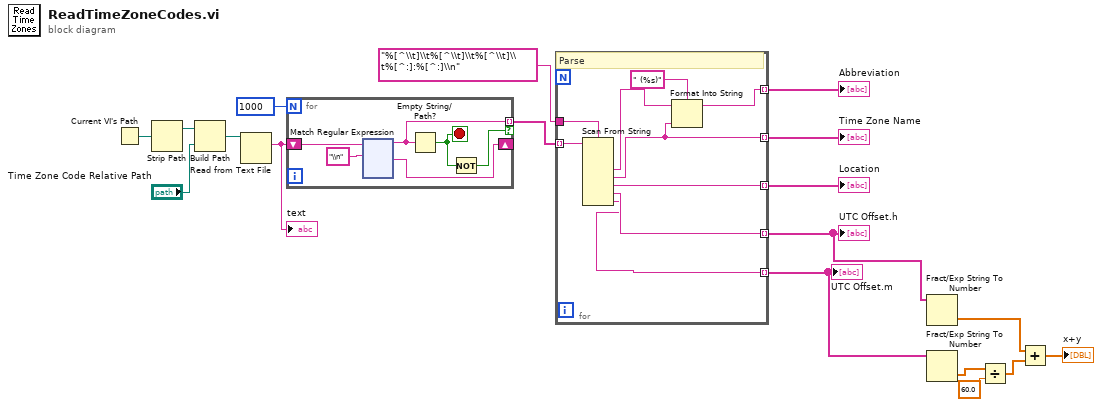
[diagram p0: block diagram]
diagram:
  n1 = Current VI's Path() -> (path=w15:path)
  n2 = Strip Path(path=w15) -> (stripped path=w14:path)  [unwired: 1 out]
  n3 = Build Path(base path=w14, name or relative path="Time Zone Code Relative Path") -> (appended path=w12:path)
  n4 = Read from Text File(file (use dialog)=w12) -> (text=w10:string)  [unwired: 3 in, 3 out]
  "text" <- w10
  n5 = for {
    N: 1000 -> [_]
    shift-right: [w22] -> _
    shift-left: w10 -> [w24]
    tunnel: [w19] -> w9 mode=indexing if=w20
    stop <- w21 stop-if-true
    # "Scan more than enough lines to get all of the Registers' string descriptions arranged into an array"
    n6 = xnode "Match Regular Expression"("input string"=w24, "regular expression"="\\n") -> ("before match"=w19:string, "after match"=w22:string)  [unwired: 4 in, 3 out]
    n7 = Empty String/Path?(string/path=w19) -> (empty?=w21:bool)
    n8 = Not(x=w21) -> (.not. x?=w20:bool)
  }
  n9 = for {
    tunnel: "%[^\\t]\\t%[^\\t]\\t%[^\\t]\\t%[^:]:%[^:]\\n" ("format string") -> [w146]
    tunnel: [w139] -> w18 mode=indexing
    tunnel: [w141] -> w16 mode=indexing
    tunnel: [w145] -> w17 mode=indexing
    tunnel: [w144] -> w7 mode=indexing
    tunnel: w9 -> [w147] mode=indexing
    tunnel: [w143] -> w6 mode=indexing
    # "Parse"
    n10 = Scan From String(format string=w146, input string=w147) -> (output 1=w142:string, output 2=w141:string, output 3=w145:string, output 4=w144:string, output 5=w143:string)  [unwired: 2 in, 8 out]
    n11 = Format Into String(format string=" (%s)", initial string=w142, w141) -> (resulting string=w139:string)  [unwired: 1 in, 1 out]
  }
  "Location" <- w17
  "UTC Offset.h" <- w7
  "Abbreviation" <- w18
  "Time Zone Name" <- w16
  "UTC Offset.m" <- w6
  n12 = Fract/Exp String To Number(string=w7) -> (number=w2:dbl[])  [unwired: 3 in, 1 out]
  n13 = Fract/Exp String To Number(string=w6) -> (number=w5:dbl[])  [unwired: 3 in, 1 out]
  n14 = Divide(x=w5, y=60.0) -> (x/y=w3:dbl[])
  n15 = Add(x=w2, y=w3) -> (x+y=→"x+y":dbl[])
